vi "calculateNextFrequency.vi"(8 "error in (no error)":errorcluster, 11 "ChirpWave in":refnum<class "ChirpWave.lvclass">) -> (0 "error out":errorcluster, 3 "ChirpWave out":refnum<class "ChirpWave.lvclass">)   [LabVIEW 2015, in "ChirpWave.lvclass"]
uses:
  ChirpWave.lvclass
  ChirpWave.lvclass/ChirpWave.ctl
  <vilib>/express/express arith-compare/Formula/XNode/ExpressFormulaBlockNode.xnode
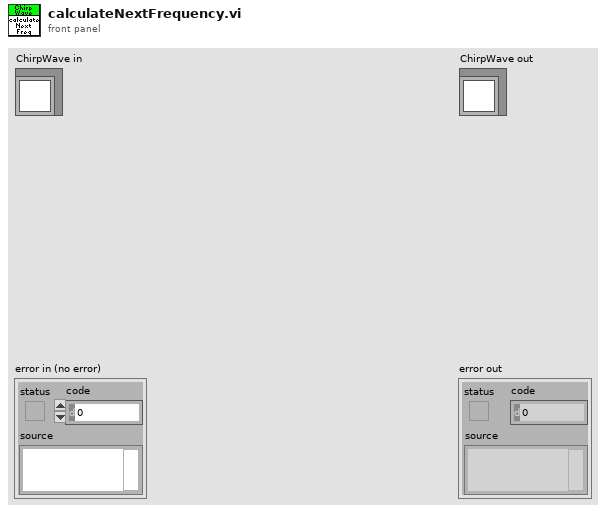
[diagram p1: front panel]
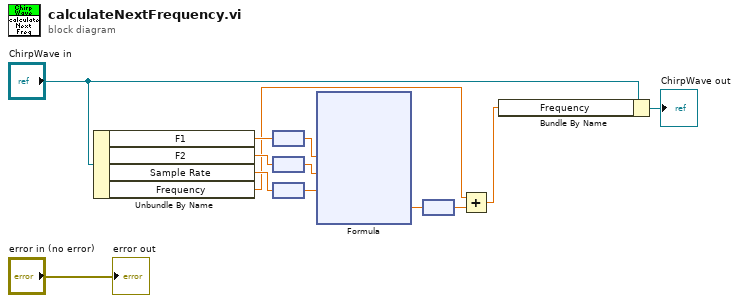
[diagram p0: block diagram]
diagram:
  n1 = Unbundle By Name("ChirpWave in") -> ("F1"=w6:dbl[unit], "F2"=w7:dbl[unit], "Sample Rate"=w10:dbl[unit], "Frequency"=w3:dbl[unit])
  n2 = node(w6) -> (w5:dbl)
  n3 = node(w7) -> (w8:dbl)
  n4 = node(w10) -> (w9:dbl)
  n5 = xnode "Formula"("F1"=w5, "F2"=w8, "RATE"=w9) -> ("Result"=w4:dbl)  [unwired: 1 in, 1 out]
  n6 = node(w4) -> (w2:dbl[unit])
  n7 = Add(x=w3, y=w2) -> (x+y=w1:dbl[unit])
  n8 = Bundle By Name(cluster="ChirpWave in", "Frequency"=w1) -> (→"ChirpWave out":refnum<class "ChirpWave.lvclass">)
  "error out" <- "error in (no error)"
